vi "Run 3.vi"(11 "EV3 in":T1) -> (3 "EV3 out":T1)   [LabVIEW 2016]
uses:
  <vilib>/NXT/Subs/LVHSConnector.ctl
  <vilib>/NXT/LegoClasses/BrickReference/BrickReference.lvclass
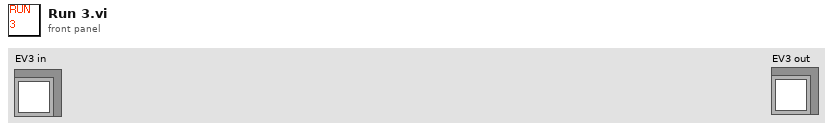
[diagram p1: front panel]
types:
  T1 = typedef "LVHSConnector.ctl" = refnum<class "BrickReference.lvclass">
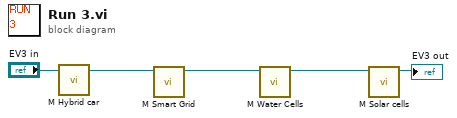
[diagram p0: block diagram]
diagram:
  n1 = call "M Hybrid car.vi"("EV3 in"="EV3 in") -> ("EV3 out"=w5:T1)  [unwired: 10 in]
  n2 = call "M Smart Grid.vi"("EV3 in"=w5) -> ("EV3 out"=w4:T1)  [unwired: 10 in]
  n3 = call "M Water Cells.vi"("EV3 in"=w4) -> ("EV3 out"=w3:T1)  [unwired: 10 in]
  n4 = call "M Solar cells.vi"("EV3 in"=w3) -> ("EV3 out"=→"EV3 out":T1)  [unwired: 10 in]
